vi "GPRS参数格式转化.vi"(1 "参数大小":u16=144, 2 "参数字符串(十进制)":string) -> (0 "参数字符串(十六进制)":string)   [LabVIEW 2015]
panel:
  # "比如\ninpt “+TU”\nout  “2b 54 55”"
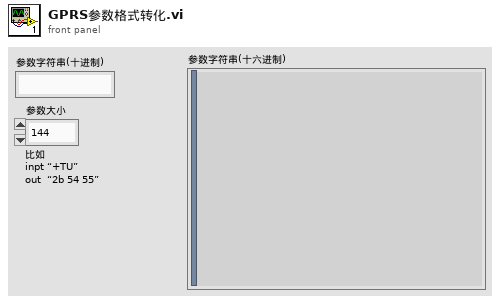
[diagram p1: front panel]
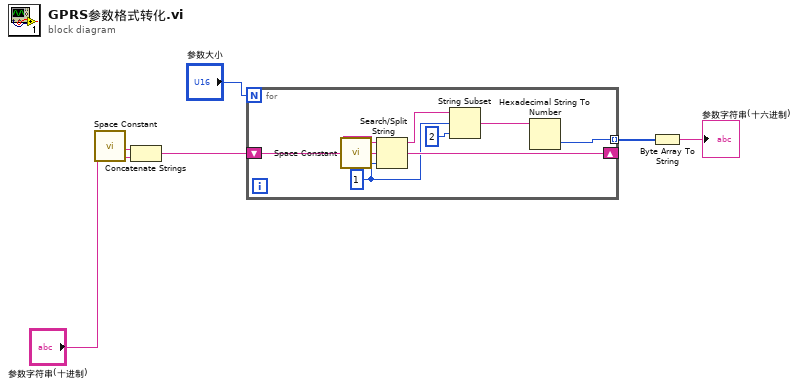
[diagram p0: block diagram]
diagram:
  n1 = call <vilib>:"Space Constant.vi"() -> ("String"=w2:string)
  n2 = Concatenate Strings(w2, "参数字符串(十进制)") -> (w5:string)
  n3 = for {
    N: "参数大小" -> [_]
    shift-right: [w13] -> _
    shift-left: w5 -> [w9]
    tunnel: [w7] -> w3 mode=indexing
    w11 = 1 ("偏移量(0)")
    n4 = call <vilib>:"Space Constant.vi"() -> ("String"=w14:string)
    n5 = Search/Split String(string=w9, search string/char (-)=w14, offset (0)=w11) -> (substring before match=w12:string, match + rest of string=w13:string)  [unwired: 1 out]
    n6 = String Subset(string=w12, offset (0)=w11, length (rest)=2 ("长度（剩余）")) -> (substring=w8:string)
    n7 = Hexadecimal String To Number(string=w8) -> (number=w7:u32)  [unwired: 2 in, 1 out]
  }
  n8 = Byte Array To String(unsigned byte array=w3) -> (string=→"参数字符串(十六进制)":string)
